vi "Agilent SNA Set RF On-Off.vi"(4 "Passthrough (T)":bool=TRUE, 7 "Agilent SNA & SWP":T1, 8 "error in (no error)":errorcluster, 10 "RF On (T)":bool=TRUE, 11 "VISA Resource Names":T2) -> (0 "error out":errorcluster, 3 "dup VISA Resource Names":T2)   [LabVIEW 2011]
doc: "This VI for the HP8753B Network Analyzers reads the stimulus values. Except when performing log sweeps and freq list sweeps, this VI uses the start and stop values and the number of points to calcuate the stimulus values."
uses:
  TypeDefs/Agilent SNA VISA.ctl
  TypeDefs/Agilent SNA Instrument Info.ctl
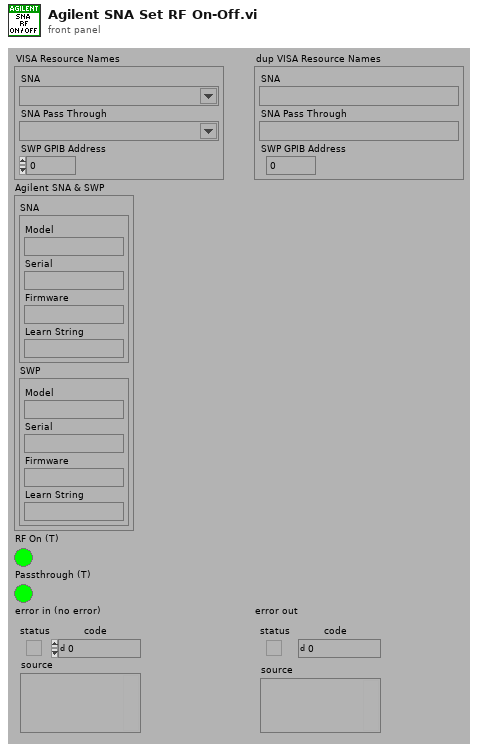
[diagram p1: front panel]
types:
  T1 = typedef "Agilent SNA Instrument Info.ctl" = cluster{"SNA":cluster{"Model":string, "Serial":string, "Firmware":string, "Learn String":string}, "SWP":cluster{"Model":string, "Serial":string, "Firmware":string, "Learn String":string}}
  T2 = typedef "Agilent SNA VISA.ctl" = cluster{"SNA":refnum<visa-resource-name>, "SNA Pass Through":refnum<visa-resource-name>, "SWP GPIB Address":i32}
  T3 = typedef "Agilent SNA Model.ctl" = enum16{"Not Supported", "8757X"}
  T4 = typedef "Agilent SNA SWP Model.ctl" = enum16{"Not Supported", "836XXX", "8375XX", "E82X7D"}
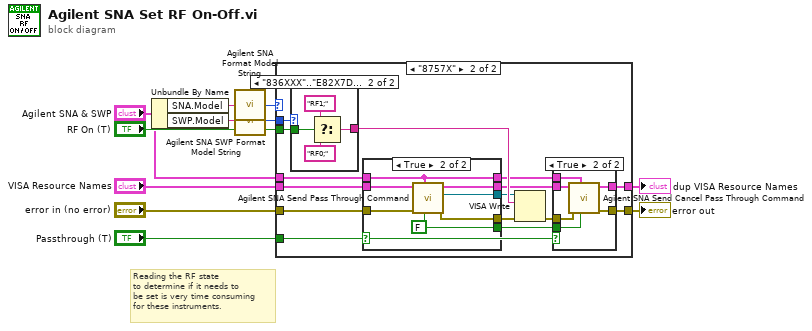
[diagram p0: block diagram]
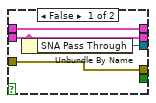
[diagram p4: hidden frame]
diagram:
  # "Reading the RF state\nto determine if it needs to\nbe set is very time consuming\nfor these instruments."
  n1 = Unbundle By Name("Agilent SNA & SWP") -> ("SNA.Model"=w8:string, "SWP.Model"=w7:string)
  n2 = call "Agilent SNA Format Model String.vi"("Model String"=w8) -> ("Model"=w6:T3)
  n3 = call "Agilent SNA SWP Format Model String.vi"("Model String"=w7) -> ("Model"=w5:T4)
  n4 = case shown="\"8757X\"" w6 {
    tunnel: [w13 w19] -> w11
    tunnel: "error in (no error)" -> [w13 w23]
    tunnel: "RF On (T)" -> [_ w27]
    tunnel: "VISA Resource Names" -> [w12 w24]
    tunnel: w5 -> [_ w26]
    tunnel: "Agilent SNA & SWP" -> [_ w25]
    tunnel: [w12 w18] -> w2
    tunnel: "Passthrough (T)" -> [_ w16]
    frame "Not Supported" {
    }
    frame "8757X" {
      n5 = case shown="\"836XXX\"..\"E82X7D\"" w26 {
        tunnel: [_ w49] -> w28
        tunnel: w27 -> [_ w48]
        frame "Not Supported" {
        }
        frame "836XXX".."E82X7D" {
          n6 = Select(t="RF1;", s=w48, f="RF0;") -> (s? t:f=w49:string)
        }
      }
      n7 = case shown="True" w16 {
        tunnel: [w39 w47] -> w22
        tunnel: w23 -> [w37 w46]
        tunnel: w24 -> [w38 w45]
        tunnel: w25 -> [w40 w42]
        tunnel: [w38 w44] -> w21
        tunnel: [_ w43] -> w15
        tunnel: [w40 w42] -> w20
        tunnel: [w37 w41] -> w14
        frame False {
          n8 = Unbundle By Name(w38) -> ("SNA Pass Through"=w39:refnum<visa-resource-name>)
        }
        frame True {
          w43 = FALSE ("SCPI? (F)")
          n9 = call "Agilent SNA Send Pass Through Command.vi"("SCPI? (F)"=w43, "Agilent SNA & SWP"=w42, "error in (no error)"=w46, "VISA Resource Names"=w45) -> ("error out"=w41:errorcluster, "SNA Pass Through"=w47:refnum<visa-resource-name>, "dup VISA Resource Names"=w44:T2)  [unwired: 5 out]
        }
      }
      n10 = VISA Write(VISA resource name=w22, write buffer=w28, error in (no error)=w14) -> (error out=w17:errorcluster)  [unwired: 2 out]
      n11 = case shown="True" w16 {
        tunnel: [w30 w36] -> w19
        tunnel: w21 -> [w29 w35]
        tunnel: w17 -> [w30 w34]
        tunnel: w15 -> [_ w33]
        tunnel: [w29 w32] -> w18
        tunnel: w20 -> [_ w31]
        frame False {
        }
        frame True {
          n12 = call "Agilent SNA Send Cancel Pass Through Command.vi"("SCPI? (F)"=w33, "Agilent SNA & SWP"=w31, "error in (no error)"=w34, "VISA Resource Names"=w35) -> ("error out"=w36:errorcluster, "dup VISA Resource Names"=w32:T2)  [unwired: 6 out]
        }
      }
    }
  }
  "dup VISA Resource Names" <- w2
  "error out" <- w11
